vi "Plus&Stay.vi"() -> (0 "s? t:f":dbl)   [LabVIEW 2014]
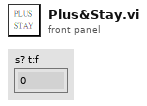
[diagram p1: front panel]
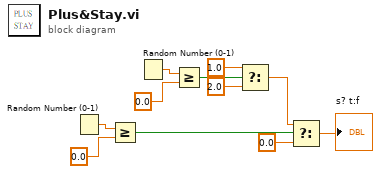
[diagram p0: block diagram]
diagram:
  n1 = Random Number (0-1)() -> (number: 0 to 1=w5:dbl)
  n2 = Greater Or Equal?(x=w5, y=0.0) -> (x >= y?=w4:bool)
  n3 = Random Number (0-1)() -> (number: 0 to 1=w11:dbl)
  n4 = Greater Or Equal?(x=w11, y=0.0) -> (x >= y?=w9:bool)
  n5 = Select(t=1.0, s=w9, f=2.0) -> (s? t:f=w2:dbl)
  n6 = Select(t=w2, s=w4, f=0.0) -> (s? t:f=→"s? t:f":dbl)
